vi "Main.vi"(8 "error in (no error)":errorcluster, 11 "AOTFBase in":refnum<class "Invivo_AOTF.lvclass">) -> (0 "error out":errorcluster, 3 "component":refnum<class "Invivo_AOTF.lvclass">)   [LabVIEW 2012, in "Invivo_AOTF.lvclass"]
doc: "Main VI of the component."
uses:
  Invivo_AOTF.lvclass
  Controls/laser line enum.ctl
  <vilib>/Distrio/Murmex/Murmex/command_enum.ctl
  Invivo_AOTF.lvclass/Invivo_AOTF.ctl
  <vilib>/Distrio/Murmex/InitialiseMessage/InitialiseMessage.lvclass
  <vilib>/Distrio/Murmex/ConfigureMessage/ConfigureMessage.lvclass
  <vilib>/Distrio/Murmex/TerminateMessage/TerminateMessage.lvclass
  <vilib>/Distrio/Murmex/Murmex/update_cluster.ctl
  <vilib>/Distrio/Murmex/GenericMessage/GenericMessage.lvclass
  <vilib>/Distrio/Murmex/Murmex/Set configure at initialise.vi
  <vilib>/Distrio/Murmex/Murmex/Set VI reference.vi
  <vilib>/Distrio/Murmex/Murmex/Get ID.vi
  <vilib>/Distrio/Murmex/Murmex/Set log reference.vi
  <vilib>/Distrio/Murmex/Message/Add or replace parameter.vi
  <vilib>/Distrio/Murmex/Murmex/Murmex.lvclass
  <vilib>/Distrio/Murmex/Message/Message.lvclass
panel:
  in  "button::configure":bool
  in  "button::quit":bool
  out "terminate?":bool=TRUE
  in  "Tab Control":enum32{"Main", "Debug"}(tab)=enum."Debug"
  in  "PowerPercentage":dbl(knob)=50.0 min=0.0 max=100.0 step=5.0 scale=0.0..100.0
  in  "button::status":bool
  in  "Line On/Off":bool
  in  "button::shutter":bool
  in  "Frequency":T1=112.075 items=["488nm"=112.08, "405nm"=150.3, "445nm"=128.71, "491nm"=110.257, "515nm"=103.5, "561nm"=93.2]
  in  "Line number":u32=1 min=1 max=8 step=1
  out "Last read buffer":string="l1F103.500P12.8S1\n\r"
  out "log":string="\r\n11:11:41.970 05/12/2013: initialise from AOTF to AOTF\r\n11:11:42.586 05/12/2013: inform from AOTF to AOTF\r\n11:11:43.913 05/12/2013: update from AOTF to AOTF\r\n11:11:45.142 05/12/2013: generic (shutter_off) from AOTF to AOTF\r\n11:11:45.270 05/12/2013: generic (shutter_on) from AOTF to AOTF\r\n11:11:45.902 05/12/2013: generic (shutter_off) from AOTF to AOTF\r\n11:11:45.932 05/12/2013: inspect from AOTF to AOTF\r\n11:11:48.013 05/12/2013: configure from AOTF to AOTF\r\n11:11:52.003 05/12/2013: inform from AOTF to AOTF\r\n11:11:58.521 05/12/2013: initialise from AOTF to AOTF\r\n11:11:58.561 05/12/2013: inform from AOTF to AOTF\r\n11:11:58.695 05/12/2013: inform from AOTF to AOTF\r\n11:12:02.089 05/12/2013: update from AOTF to AOTF\r\n11:12:02.308 05/12/2013: inspect from AOTF to AOTF\r\n11:12:02.364 05/12/2013: inform from AOTF to AOTF\r\n11:12:05.062 05/12/2013: generic (shutter_on) from AOTF to AOTF\r\n11:12:06.690 05/12/2013: update from AOTF to AOTF\r\n11:12:06.909 05/12/2013: inspect from AOTF to AOTF\r\n11:12:06.964 05/12/2013: inform from AOTF to AOTF\r\n11:12:07.770 05/12/2013: update from AOTF to AOTF\r\n11:12:07.989 05/12/2013: inspect from AOTF to AOTF\r\n11:12:08.044 05/12/2013: inform from AOTF to AOTF\r\n11:12:08.627 05/12/2013: update from AOTF to AOTF\r\n11:12:08.846 05/12/2013: inspect from AOTF to AOTF\r\n11:12:08.900 05/12/2013: inform from AOTF to AOTF\r\n11:12:09.290 05/12/2013: update from AOTF to AOTF\r\n11:12:09.508 05/12/2013: inspect from AOTF to AOTF\r\n11:12:09.563 05/12/2013: inform from AOTF to AOTF\r\n11:12:10.154 05/12/2013: update from AOTF to AOTF\r\n11:12:10.373 05/12/2013: inspect from AOTF to AOTF\r\n11:12:10.430 05/12/2013: inform from AOTF to AOTF\r\n11:12:20.953 05/12/2013: update from AOTF to AOTF\r\n11:12:21.172 05/12/2013: inspect from AOTF to AOTF\r\n11:12:21.227 05/12/2013: inform from AOTF to AOTF\r\n11:12:22.057 05/12/2013: update from AOTF to AOTF\r\n11:12:22.276 05/12/2013: inspect from AOTF to AOTF\r\n11:12:22.330 05/12/2013: inform from AOTF to AOTF\r\n11:12:22.841 05/12/2013: update from AOTF to AOTF\r\n11:12:23.060 05/12/2013: inspect from AOTF to AOTF\r\n11:12:23.114 05/12/2013: inform from AOTF to AOTF\r\n11:12:23.449 05/12/2013: update from AOTF to AOTF\r\n11:12:23.668 05/12/2013: inspect from AOTF to AOTF\r\n11:12:23.724 05/12/2013: inform from AOTF to AOTF\r\n11:12:24.514 05/12/2013: update from AOTF to AOTF\r\n11:12:24.733 05/12/2013: inspect from AOTF to AOTF\r\n11:12:24.789 05/12/2013: inform from AOTF to AOTF\r\n11:12:25.098 05/12/2013: update from AOTF to AOTF\r\n11:12:25.317 05/12/2013: inspect from AOTF to AOTF\r\n11:12:25.371 05/12/2013: inform from AOTF to AOTF\r\n11:12:26.482 05/12/2013: update from AOTF to AOTF\r\n11:12:26.701 05/12/2013: inspect from AOTF to AOTF\r\n11:12:26.755 05/12/2013: inform from AOTF to AOTF\r\n11:12:27.154 05/12/2013: update from AOTF to AOTF\r\n11:12:27.373 05/12/2013: inspect from AOTF to AOTF\r\n11:12:27.428 05/12/2013: inform from AOTF to AOTF\r\n11:12:27.666 05/12/2013: update from AOTF to AOTF\r\n11:12:27.885 05/12/2013: inspect from AOTF to AOTF\r\n11:12:27.944 05/12/2013: inform from AOTF to AOTF\r\n11:12:33.380 05/12/2013: update from AOTF to AOTF\r\n11:12:33.484 05/12/2013: update from AOTF to AOTF\r\n11:12:33.603 05/12/2013: inspect from AOTF to AOTF\r\n11:12:33.611 05/12/2013: update from AOTF to AOTF\r\n11:12:33.684 05/12/2013: update from AOTF to AOTF\r\n11:12:33.740 05/12/2013: update from AOTF to AOTF\r\n11:12:33.827 05/12/2013: inspect from AOTF to AOTF\r\n11:12:33.835 05/12/2013: update from AOTF to AOTF\r\n11:12:33.897 05/12/2013: inform from AOTF to AOTF\r\n11:12:33.903 05/12/2013: update from AOTF to AOTF\r\n11:12:33.940 05/12/2013: update from AOTF to AOTF\r\n11:12:34.085 05/12/2013: update from AOTF to AOTF\r\n11:12:34.119 05/12/2013: inspect from AOTF to AOTF\r\n11:12:34.292 05/12/2013: update from AOTF to AOTF\r\n11:12:34.336 05/12/2013: inspect from AOTF to AOTF\r\n11:12:34.553 05/12/2013: inspect from AOTF to AOTF\r\n11:12:34.608 05/12/2013: inform from AOTF to AOTF\r\n11:12:34.739 05/12/2013: update from AOTF to AOTF\r\n11:12:34.771 05/12/2013: update from AOTF to AOTF\r\n11:12:34.826 05/12/2013: inspect from AOTF to AOTF\r\n11:12:34.834 05/12/2013: update from AOTF to AOTF\r\n11:12:34.867 05/12/2013: update from AOTF to AOTF\r\n11:12:34.931 05/12/2013: update from AOTF to AOTF\r\n11:12:34.979 05/12/2013: update from AOTF to AOTF\r\n11:12:35.003 05/12/2013: update from AOTF to AOTF\r\n11:12:35.027 05/12/2013: update from AOTF to AOTF\r\n11:12:35.041 05/12/2013: update from AOTF to AOTF\r\n11:12:35.051 05/12/2013: inspect from AOTF to AOTF\r\n11:12:35.066 05/12/2013: update from AOTF to AOTF\r\n11:12:35.116 05/12/2013: update from AOTF to AOTF\r\n11:12:35.171 05/12/2013: update from AOTF to AOTF\r\n11:12:35.211 05/12/2013: update from AOTF to AOTF\r\n11:12:35.273 05/12/2013: inspect from AOTF to AOTF\r\n11:12:35.287 05/12/2013: update from AOTF to AOTF\r\n11:12:35.475 05/12/2013: update from AOTF to AOTF\r\n11:12:35.495 05/12/2013: inspect from AOTF to AOTF\r\n11:12:35.549 05/12/2013: inform from AOTF to AOTF\r\n11:12:35.764 05/12/2013: inspect from AOTF to AOTF\r\n11:12:35.819 05/12/2013: inform from AOTF to AOTF\r\n11:12:35.861 05/12/2013: update from AOTF to AOTF\r\n11:12:35.877 05/12/2013: inform from AOTF to AOTF\r\n11:12:35.947 05/12/2013: update from AOTF to AOTF\r\n11:12:36.067 05/12/2013: update from AOTF to AOTF\r\n11:12:36.100 05/12/2013: inspect from AOTF to AOTF\r\n11:12:36.235 05/12/2013: update from AOTF to AOTF\r\n11:12:36.317 05/12/2013: inspect from AOTF to AOTF\r\n11:12:36.371 05/12/2013: inform from AOTF to AOTF\r\n11:12:36.587 05/12/2013: inspect from AOTF to AOTF\r\n11:12:36.771 05/12/2013: update from AOTF to AOTF\r\n11:12:36.804 05/12/2013: inspect from AOTF to AOTF\r\n11:12:37.020 05/12/2013: inspect from AOTF to AOTF\r\n11:12:37.238 05/12/2013: inspect from AOTF to AOTF\r\n11:12:37.456 05/12/2013: inspect from AOTF to AOTF\r\n11:12:37.673 05/12/2013: inspect from AOTF to AOTF\r\n11:12:37.891 05/12/2013: inspect from AOTF to AOTF\r\n11:12:37.946 05/12/2013: inform from AOTF to AOTF\r\n11:12:38.161 05/12/2013: inspect from AOTF to AOTF\r\n11:12:38.379 05/12/2013: inspect from AOTF to AOTF\r\n11:12:38.597 05/12/2013: inspect from AOTF to AOTF\r\n11:12:38.815 05/12/2013: inspect from AOTF to AOTF\r\n11:12:38.871 05/12/2013: inform from AOTF to AOTF\r\n11:12:39.086 05/12/2013: inspect from AOTF to AOTF\r\n11:12:39.303 05/12/2013: inspect from AOTF to AOTF\r\n11:12:39.363 05/12/2013: inform from AOTF to AOTF\r\n11:12:39.417 05/12/2013: inform from AOTF to AOTF\r\n11:12:39.633 05/12/2013: inspect from AOTF to AOTF\r\n11:12:39.852 05/12/2013: inspect from AOTF to AOTF\r\n11:12:40.069 05/12/2013: inspect from AOTF to AOTF\r\n11:12:40.124 05/12/2013: inform from AOTF to AOTF\r\n11:12:40.339 05/12/2013: inspect from AOTF to AOTF\r\n11:12:40.395 05/12/2013: inform from AOTF to AOTF\r\n11:12:40.448 05/12/2013: inform from AOTF to AOTF\r\n11:12:40.663 05/12/2013: inspect from AOTF to AOTF\r\n11:12:40.718 05/12/2013: inform from AOTF to AOTF\r\n11:12:40.770 05/12/2013: inform from AOTF to AOTF\r\n11:12:40.824 05/12/2013: inform from AOTF to AOTF\r\n11:12:40.877 05/12/2013: inform from AOTF to AOTF\r\n11:12:40.930 05/12/2013: inform from AOTF to AOTF\r\n11:12:40.982 05/12/2013: inform from AOTF to AOTF\r\n11:12:41.034 05/12/2013: inform from AOTF to AOTF\r\n11:12:41.092 05/12/2013: inform from AOTF to AOTF\r\n11:12:41.144 05/12/2013: inform from AOTF to AOTF\r\n11:12:41.196 05/12/2013: inform from AOTF to AOTF\r\n11:12:41.249 05/12/2013: inform from AOTF to AOTF\r\n11:12:41.307 05/12/2013: inform from AOTF to AOTF\r\n11:12:41.366 05/12/2013: inform from AOTF to AOTF\r\n11:12:41.424 05/12/2013: inform from AOTF to AOTF\r\n11:12:41.478 05/12/2013: inform from AOTF to AOTF\r\n11:12:41.533 05/12/2013: inform from AOTF to AOTF\r\n11:12:41.589 05/12/2013: inform from AOTF to AOTF\r\n11:12:42.246 05/12/2013: terminate from AOTF to AOTF"
  in  "component ID":string="AOTF"
  in  "button::send":bool
  in  "command":T2
  in  "Generic command":string
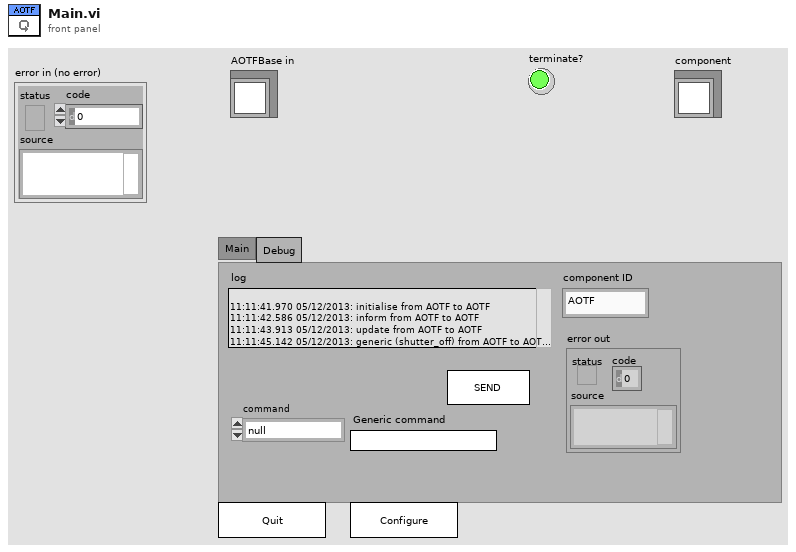
[diagram p1: front panel]
types:
  T1 = typedef "Invivo_AOTF.lvclass/laser line enum.ctl" = dbl
  T2 = typedef "Murmex.lvlib/Murmex.lvclass/command_enum.ctl" = enum16{"null", "initialise", "reset", "terminate", "acknowledge", "update", "inspect", "inform", "proceed", "start", "stop", "fetch", "configure", "generic"}
  T3 = enum8{"Enabled", "Disabled", "Disabled and Grayed Out"}
  T4 = typedef "Murmex.lvlib/Murmex.lvclass/update_cluster.ctl" = cluster{"target ID":string, "key chains":string[], "values":variant[]}
  T5 = typedef "Murmex.lvclass/command_enum.ctl" = enum16{"null", "initialise", "reset", "terminate", "acknowledge", "update", "inspect", "inform", "proceed", "start", "stop", "fetch", "configure", "generic"}
  T6 = typedef "Murmex.lvclass/Event type enumerations.ctl" = enum16{"before", "after"}
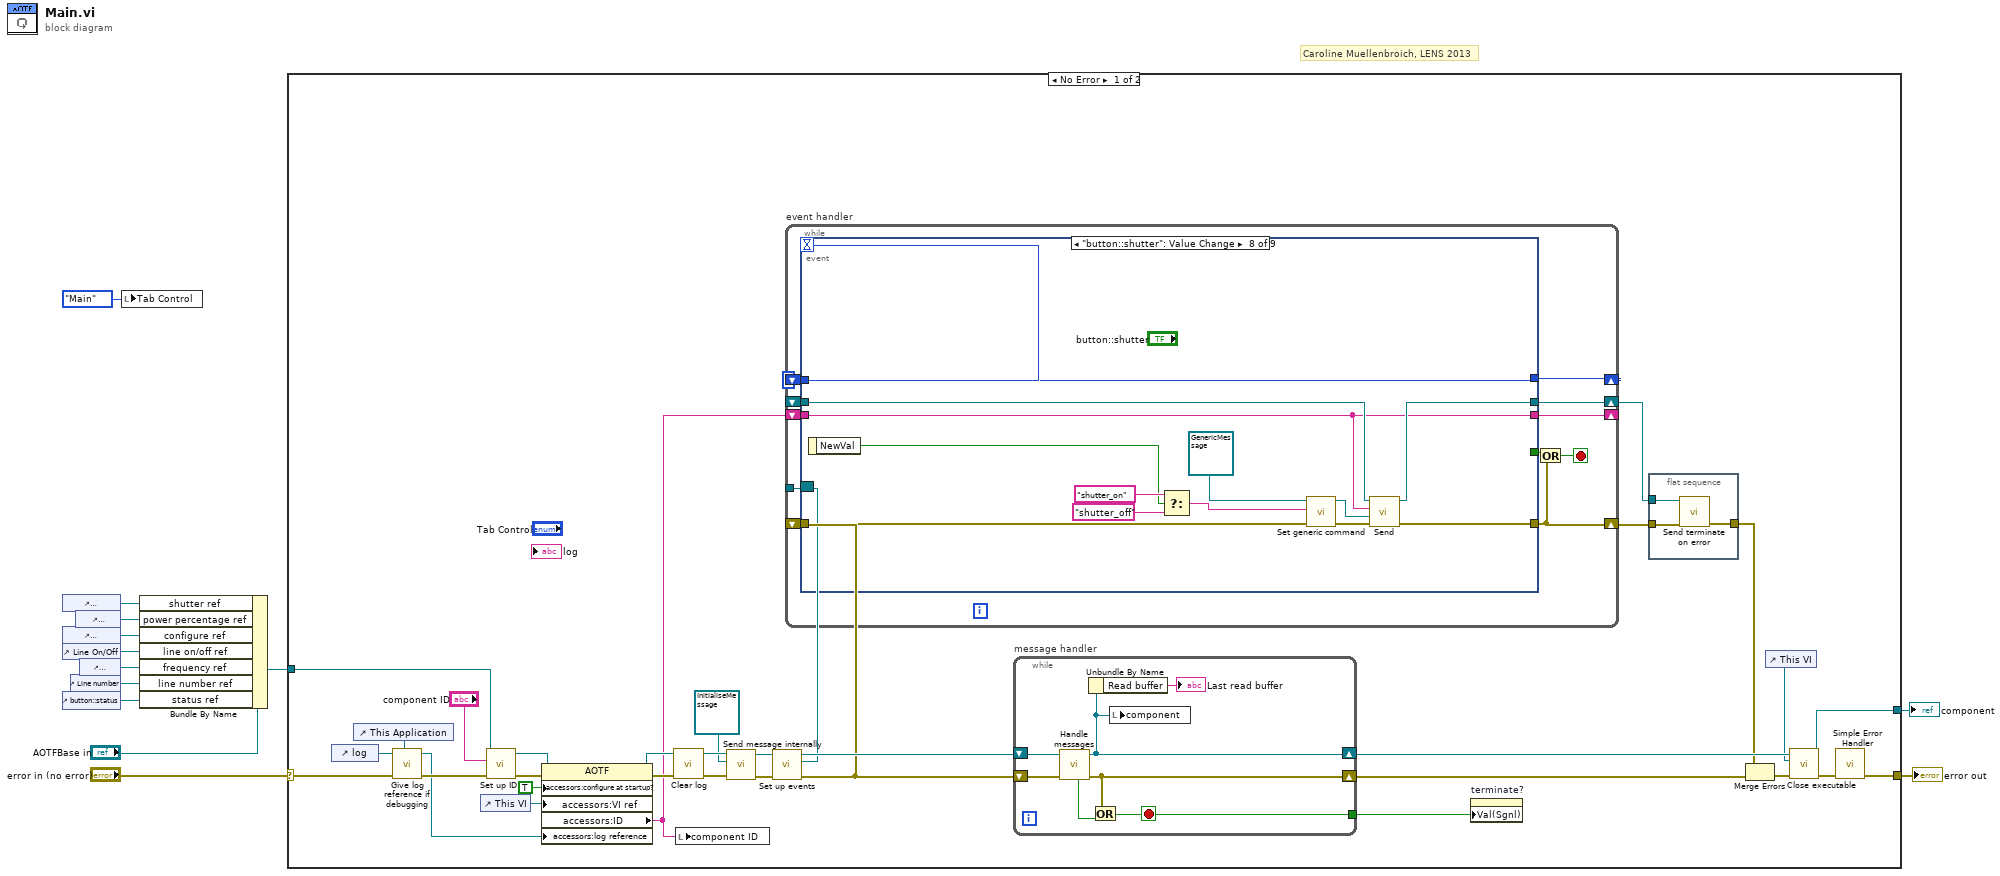
[diagram p0: block diagram]
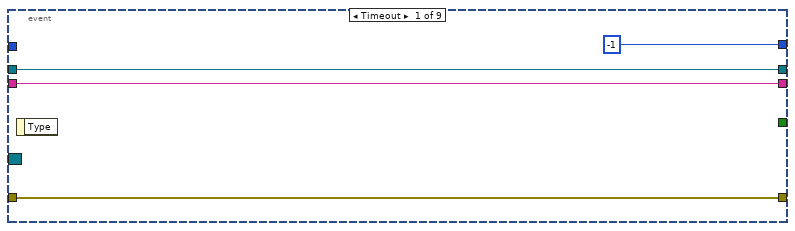
[diagram p2: hidden frame]
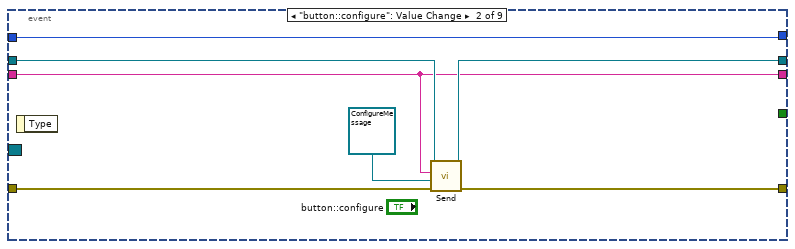
[diagram p3: hidden frame]
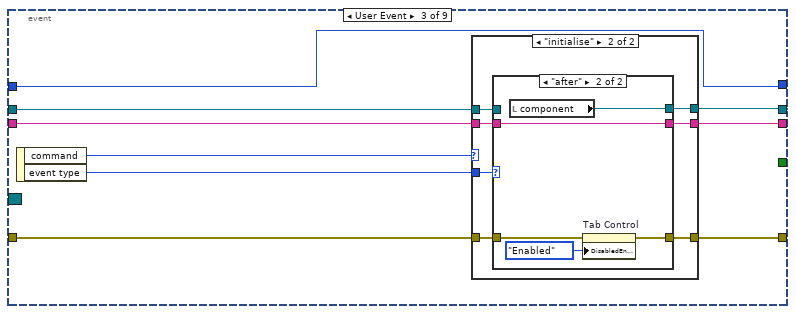
[diagram p4: hidden frame]
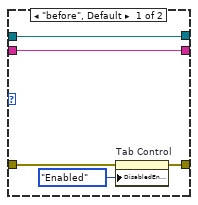
[diagram p6: hidden frame]
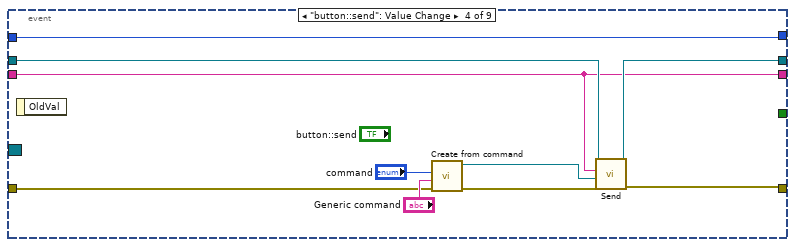
[diagram p7: hidden frame]
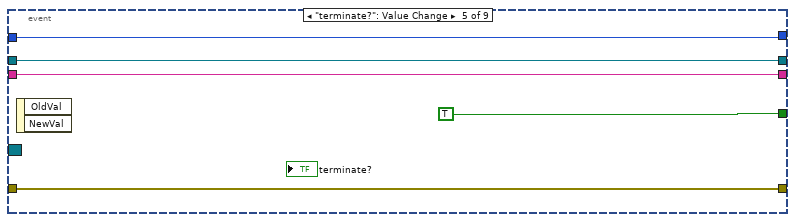
[diagram p8: hidden frame]
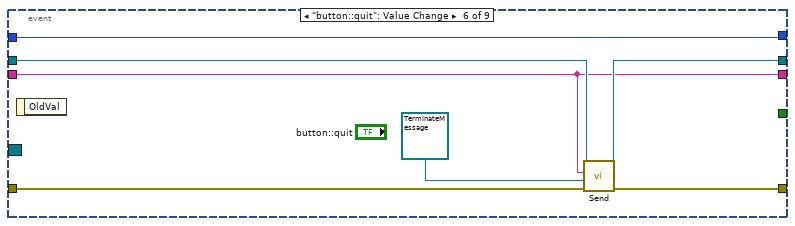
[diagram p9: hidden frame]
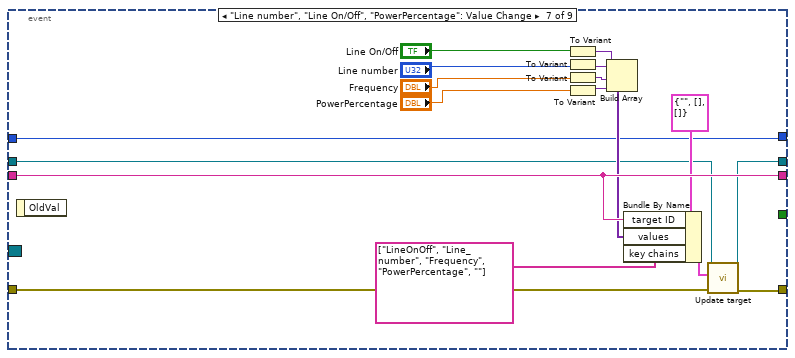
[diagram p10: hidden frame]
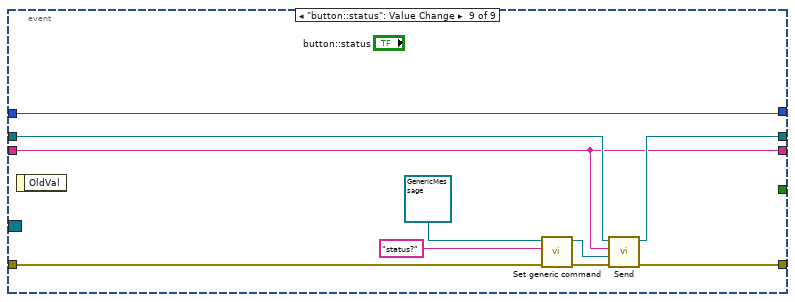
[diagram p11: hidden frame]
diagram:
  # "Caroline Muellenbroich, LENS 2013"
  n1 = control-ref of="button::shutter"() -> (w4:refnum<vi>)
  n2 = control-ref of="button::configure"() -> (w7:refnum<vi>)
  n3 = control-ref of="Line On/Off"() -> (w2:refnum<vi>)
  n4 = control-ref of="button::status"() -> (w1:refnum<vi>)
  n5 = control-ref of="Line number"() -> (w5:refnum<vi>)
  n6 = control-ref of="PowerPercentage"() -> (w3:refnum<vi>)
  n7 = control-ref of="Frequency"() -> (w6:refnum<vi>)
  n8 = local write "Tab Control"(enum32{"Main", "Debug"}."Main" ("Tab Control")) -> ()
  n9 = Bundle By Name(cluster="AOTFBase in", "shutter ref"=w4, "power percentage ref"=w3, "configure ref"=w7, "line on/off ref"=w2, "frequency ref"=w6, "line number ref"=w5, "status ref"=w1) -> (w8:refnum<class "Invivo_AOTF.lvclass">)
  n10 = case shown="No Error" "error in (no error)" {
    selector: "error in (no error)" -> [w16 w173]
    tunnel: w8 -> [w47 w172]
    tunnel: [w31 w172] -> w13
    tunnel: [w27 w173] -> w12
    frame No Error {
      n11 = control-ref of="log"() -> (w17:refnum<vi>)
      n12 = control-ref of="This Application"() -> (w18:refnum<vi>)
      n13 = call "Give log reference if debugging.vi"("application ref"=w18, "error in (no error)"=w16, "log reference in"=w17) -> ("error out"=w15:errorcluster, "log reference out"=w14:refnum<vi>)  [unwired: 6 in, 1 out]
      n14 = control-ref of="This VI"() -> (w43:refnum<vi>)
      n15 = call <vilib>:"Set up ID.vi"("error in (no error)"=w15, "component ID"="component ID", "MurmexBase in"=w47) -> ("error out"=w46:errorcluster, "MurmexBase out"=w45:refnum<class "Invivo_AOTF.lvclass">)  [unwired: 6 in, 1 out]
      n16 = property class="AOTF"(reference=w45, error in=w46, "accessors:configure at startup?"=TRUE ("configure at startup?"), "accessors:VI ref"=w43, "accessors:log reference"=w14) -> (reference out=w40:refnum<class "Invivo_AOTF.lvclass">, error out=w42:errorcluster, "accessors:ID"=w21:string)
      n17 = call <vilib>:"Clear log.vi"("error in (no error)"=w42, "MurmexBase in"=w40) -> ("error out"=w41:errorcluster, "MurmexBase out"=w39:refnum<class "Invivo_AOTF.lvclass">)  [unwired: 8 in]
      n18 = local write "component ID"(w21) -> ()
      n19 = call <vilib>:"Send message internally.vi"("error in (no error)"=w41, "Message"=refnum<class "InitialiseMessage.lvclass"> refnum ("Murmex.lvlib:InitialiseMessage"), "Murmex in"=w39) -> ("error out"=w38:errorcluster, "Murmex out"=w37:refnum<class "Invivo_AOTF.lvclass">)  [unwired: 7 in]
      n20 = call <vilib>:"Set up events.vi"("error in (no error)"=w38, "MurmexBase in"=w37) -> ("error out"=w30:errorcluster, "Event Registration Refnum"=w29:refnum<event-registration>, "MurmexBase out"=w36:refnum<class "Invivo_AOTF.lvclass">)  [unwired: 7 in]
      n21 = while "event handler" {
        tunnel: w29 -> [w61]
        shift-right: [w54] -> w25
        shift-left: w30 -> [w60]
        shift-right: [w56] -> _
        shift-left: w21 -> [w59]
        shift-right: [w58] -> w23
        shift-left: _ -> [w57]
        shift-right: [w52] -> _
        shift-left: 0 -> [w51]
        stop <- w55 stop-if-true
        n22 = event shown="[7] \"button::shutter\": Value Change" {
          selector: w61 -> [_ _ _ _ _ _ _ _ _]
          dyn-events: _ -> [_ _ _ _ _ _ _ _ _]
          timeout: w51 -> [_ _ _ _ _ _ _ _ _]
          tunnel: w60 -> [w63 w72 w79 w108 w116 w123 w140 w152 w162]
          tunnel: [w63 w71 w78 w107 w116 w122 w141 w153 w163] -> w54
          tunnel: w59 -> [w65 w67 w77 w103 w114 w118 w139 w145 w157]
          tunnel: [w64 w69 w76 w105 w113 w120 w133 w149 w159] -> w58
          tunnel: w57 -> [w64 w70 w75 w106 w113 w121 w134 w150 w160]
          tunnel: [w65 w67 w74 w103 w114 w118 w139 w145 w157] -> w56
          tunnel: [_ _ _ _ TRUE _ _ _ _] -> w53
          tunnel: w51 -> [_ w68 w73 w104 w112 w119 w126 w143 w156]
          tunnel: [-1 w68 w73 w104 w112 w119 w126 w143 w156] -> w52
          event Timeout {
            n23 = event-data() -> ()  [unwired: 1 in, 1 out]
          }
          event "button::configure": Value Change {
            n24 = event-data() -> ()  [unwired: 1 in, 1 out]
            n25 = call <vilib>:"Send.vi"("error in (no error)"=w72, "Message"=refnum<class "ConfigureMessage.lvclass"> refnum ("Murmex.lvlib:ConfigureMessage"), "recipient"=w67, "Murmex in"=w70) -> ("error out"=w71:errorcluster, "Murmex out"=w69:refnum<class "Murmex.lvclass">)  [unwired: 6 in]
          }
          event User Event {
            n26 = event-data() -> ("command"=w81:T5, "event type"=w80:T6)  [unwired: 1 in]
            n27 = case shown="\"initialise\"" w81 {
              tunnel: w80 -> [_ w91]
              tunnel: w79 -> [w82 w90]
              tunnel: [w82 w89] -> w78
              tunnel: w77 -> [w84 w88]
              tunnel: [w83 w87] -> w76
              tunnel: w75 -> [w83 w86]
              tunnel: [w84 w85] -> w74
              frame "null", Default {
              }
              frame "initialise" {
                n28 = case shown="\"after\"" w91 {
                  tunnel: [w95 w100] -> w89
                  tunnel: w90 -> [w96 w101]
                  tunnel: w88 -> [w93 w97]
                  tunnel: [w92 w99] -> w87
                  tunnel: w86 -> [w92 _]
                  tunnel: [w93 w97] -> w85
                  frame "before", Default {
                    n29 = property on="Tab Control" class="TabCtl (strict)"(error in=w96, "DisabledEnum"=T3."Enabled" ("Disabled")) -> (error out=w95:errorcluster)  [unwired: 1 in, 1 out]
                  }
                  frame "after" {
                    n30 = local read "component"() -> (w99:refnum<class "Invivo_AOTF.lvclass">)
                    n31 = property on="Tab Control" class="TabCtl (strict)"(error in=w101, "DisabledEnum"=T3."Enabled" ("Disabled")) -> (error out=w100:errorcluster)  [unwired: 1 in, 1 out]
                  }
                }
              }
            }
          }
          event "button::send": Value Change {
            n32 = event-data() -> ()  [unwired: 1 in, 1 out]
            n33 = call <vilib>:"Create from command.vi"("error in (no error)"=w108, "generic command"="Generic command", "command"="command") -> ("error out"=w110:errorcluster, "Message out"=w109:refnum<class "Message.lvclass">)  [unwired: 7 in]
            n34 = call <vilib>:"Send.vi"("error in (no error)"=w110, "Message"=w109, "recipient"=w103, "Murmex in"=w106) -> ("error out"=w107:errorcluster, "Murmex out"=w105:refnum<class "Murmex.lvclass">)  [unwired: 6 in]
          }
          event "terminate?": Value Change {
            n35 = event-data() -> ()  [unwired: 1 in, 2 out]
          }
          event "button::quit": Value Change {
            n36 = event-data() -> ()  [unwired: 1 in, 1 out]
            n37 = call <vilib>:"Send.vi"("error in (no error)"=w123, "Message"=refnum<class "TerminateMessage.lvclass"> refnum ("Murmex.lvlib:TerminateMessage"), "recipient"=w118, "Murmex in"=w121) -> ("error out"=w122:errorcluster, "Murmex out"=w120:refnum<class "Murmex.lvclass">)  [unwired: 6 in]
          }
          event "Line number", "Line On/Off", "PowerPercentage": Value Change {
            n38 = event-data() -> ()  [unwired: 1 in, 1 out]
            n39 = To Variant(anything="Line On/Off") -> (Variant=w132:variant)
            n40 = To Variant(anything="Line number") -> (Variant=w129:variant)
            n41 = To Variant(anything="Frequency") -> (Variant=w130:variant)
            n42 = To Variant(anything="PowerPercentage") -> (Variant=w131:variant)
            n43 = Build Array(w132, w129, w130, w131) -> (w135:variant[])
            n44 = Bundle By Name(cluster=T4 {"target ID"="", "key chains"=[], "values"=[]} ("update cluster"), "target ID"=w139, "values"=w135, "key chains"=string[] ["LineOnOff", "Line_number", "Frequency", "PowerPercentage", ""]) -> (w138:T4)
            n45 = call <vilib>:"Update target.vi"("error in (no error)"=w140, "update cluster"=w138, "MurmexBase in"=w134) -> ("error out"=w141:errorcluster, "MurmexBase out"=w133:refnum<class "Murmex.lvclass">)  [unwired: 7 in]
          }
          event "button::shutter": Value Change {
            n46 = event-data() -> ("NewVal"=w144:bool)  [unwired: 1 in]
            n47 = Select(t="shutter_on" ("generic command"), s=w144, f="shutter_off" ("generic command")) -> (s? t:f=w146:string)
            n48 = call <vilib>:"Set generic command.vi"("error in (no error)"=w152, "generic command"=w146, "GenericMessage in"=refnum<class "GenericMessage.lvclass"> refnum ("Murmex.lvlib:GenericMessage")) -> ("error out"=w151:errorcluster, "GenericMessage out"=w154:refnum<class "GenericMessage.lvclass">)  [unwired: 7 in]
            n49 = call <vilib>:"Send.vi"("error in (no error)"=w151, "Message"=w154, "recipient"=w145, "Murmex in"=w150) -> ("error out"=w153:errorcluster, "Murmex out"=w149:refnum<class "Murmex.lvclass">)  [unwired: 6 in]
          }
          event "button::status": Value Change {
            n50 = event-data() -> ()  [unwired: 1 in, 1 out]
            n51 = call <vilib>:"Set generic command.vi"("error in (no error)"=w162, "generic command"="status?", "GenericMessage in"=refnum<class "GenericMessage.lvclass"> refnum ("Murmex.lvlib:GenericMessage")) -> ("error out"=w161:errorcluster, "GenericMessage out"=w164:refnum<class "GenericMessage.lvclass">)  [unwired: 7 in]
            n52 = call <vilib>:"Send.vi"("error in (no error)"=w161, "Message"=w164, "recipient"=w157, "Murmex in"=w160) -> ("error out"=w163:errorcluster, "Murmex out"=w159:refnum<class "Murmex.lvclass">)  [unwired: 6 in]
          }
        }
        n53 = Or(x=w53, y=w54) -> (x .or. y?=w55:bool)
      }
      n54 = while "message handler" {
        shift-right: [w166] -> w32
        shift-left: w36 -> [w170]
        shift-right: [w169] -> w33
        shift-left: w30 -> [w171]
        tunnel: [w167] -> w28
        stop <- w167 stop-if-true
        n55 = call <vilib>:"Handle messages.vi"("error in (no error)"=w171, "Murmex in"=w170) -> ("error out"=w169:errorcluster, "Murmex out"=w166:refnum<class "Invivo_AOTF.lvclass">, "terminated?"=w168:bool)  [unwired: 7 in]
        n56 = Unbundle By Name(w166) -> ("Read buffer"=→"Last read buffer":string)
        n57 = Or(x=w169, y=w168) -> (x .or. y?=w167:bool)
        n58 = local write "component"(w166) -> ()
      }
      n59 = property on="terminate?" class="Bool (strict)"("Val(Sgnl)"=w28) -> ()  [unwired: 2 in, 2 out]
      n60 = flat-sequence {
        tunnel: w25 -> [w49]
        tunnel: [w50] -> w24
        tunnel: w23 -> [w48]
        frame #0 {
          n61 = call <vilib>:"Send terminate on error.vi"("error in (no error)"=w49, "Murmex in"=w48) -> ("error out"=w50:errorcluster)  [unwired: 8 in, 1 out]
        }
      }
      n62 = Merge Errors(w24, w33) -> (w34:errorcluster)
      n63 = control-ref of="This VI"() -> (w22:refnum<vi>)
      n64 = call <vilib>:"Close executable.vi"("error in (no error)"=w34, "main VI ref (optional)"=w22, "MurmexBase in"=w32) -> ("error out"=w35:errorcluster, "MurmexBase out"=w31:refnum<class "Invivo_AOTF.lvclass">)  [unwired: 7 in]
      n65 = call <vilib>:"Simple Error Handler.vi"("error in (no error)"=w35) -> ("error out"=w27:errorcluster)  [unwired: 4 in, 4 out]
    }
    frame Error {
    }
  }
  "error out" <- w12
  "component" <- w13
